vi "Reverse PS_Settings.vi"(10 "Array In":T1[](array[typedef])) -> (2 "Array Out":T1[](array[typedef]))   [LabVIEW 2015]
uses:
  PS_Settings.ctl
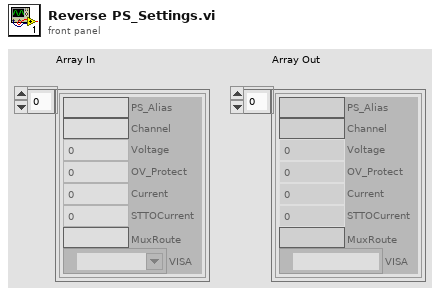
[diagram p1: front panel]
types:
  T1 = typedef "PS_Settings.ctl" = cluster{"PS_Alias":string, "Channel":string, "Voltage":dbl, "OV_Protect":dbl, "Current":dbl, "STTOCurrent":dbl, "MuxRoute":string, "VISA":refnum<visa-resource-name>}
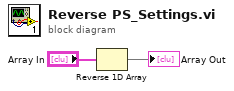
[diagram p0: block diagram]
diagram:
  n1 = Reverse 1D Array(array="Array In") -> (reversed array=→"Array Out":T1[])
